vi "Test Open Close.vi"(8 "error in (no error)":errorcluster, 11 "Instrument.Oxford1820 in":refnum<class "Instrument.OxfordVRM.lvclass">) -> (0 "error out":errorcluster, 3 "Instrument.Oxford1820 out":refnum<class "Instrument.OxfordVRM.lvclass">)   [LabVIEW 2019, in "Instrument.OxfordVRM.lvclass"]
uses:
  Instrument.OxfordVRM.lvclass
  <instrlib>/Mercury iXX/Public/Libraries/Magnet/Controls/Device (Read).ctl
  <instrlib>/Mercury iXX/Public/Controls/Manufacturing Data.ctl
  <instrlib>/Mercury iXX/Public/Libraries/Magnet/Controls/Signals (Read).ctl
  Instrument.OxfordVRM.lvclass/Instrument.OxfordVRM.ctl
  <instrlib>/Mercury iXX/Public/Libraries/Magnet/Open/Open Magnet Device.vi
  <instrlib>/Mercury iXX/Public/Libraries/Magnet/Configuration/Read/Magnet Device (Read).vi
  <instrlib>/Mercury iXX/Mercury iXX.lvlib
  <instrlib>/Mercury iXX/Public/Libraries/Magnet.lvlib
panel:
  out "Magnet Device Details":T1={"Manufacturing"={"Hardware Version"="", "Firmware Version"="", "Serial Number"=""}, "Nickname"="", "Bipolar Output"="", "String"="SERS", "Current Limit"=0.0, "AtoB"=0.0, "Inductance"=0.0, "Switch Present"="", "Swh Htr Current"=0.0, "SW VLIM"=0.0, "V Trans Time"=0.0, "Magnet PSU Signals"={"Voltage"=0.0, "Current"=0.0, "Current Rate"=0.0, "Field"=0.0, "Field Rate"=0.0, "Persistant Current"=0.0, "Persistant Field"=0.0, "Target Current"=0.0, "Target Field"=0.0, "Target Current Rate"=0.0, "Target Field Rate"=0.0, "Switch Heater Status (SWHT)"="", "Switch Heater Status (SWHN)"=""}, "PSU Action"="SERS", "Status"="", "Level Limit"=0.0, "Temperature Limit"=0.0} {"Temperature Limit" format="%#.1f"; "Level Limit" format="%#.1f"; "V Trans Time" format="%#.1f"; "SW VLIM" format="%#.1f"; "Swh Htr Current" format="%#.1f"; "Inductance" format="%#.1f"; "AtoB" format="%#.1f"; "Current Limit" format="%#.1f"}
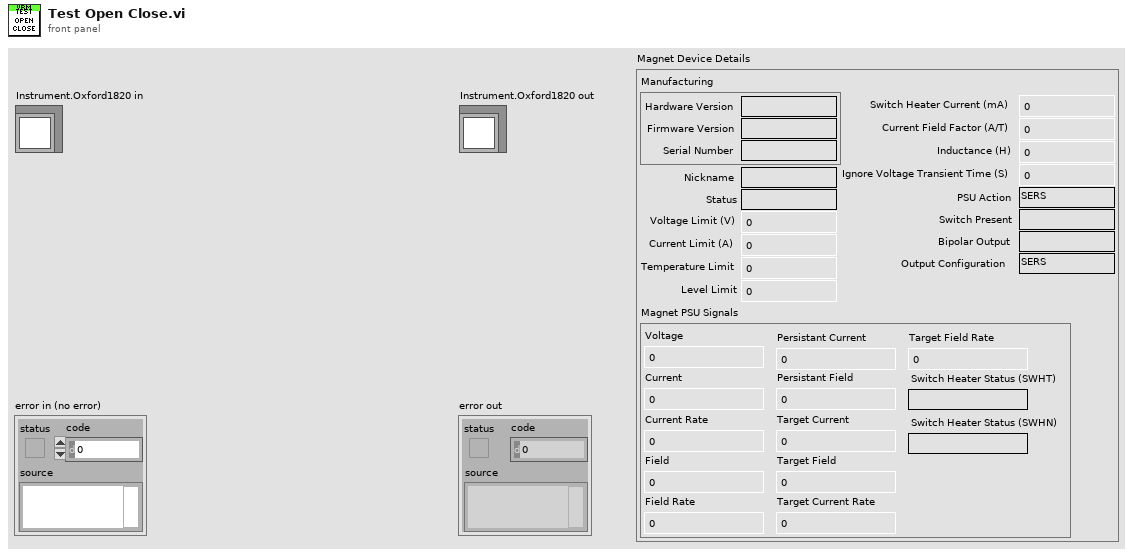
[diagram p1: front panel]
types:
  T1 = typedef "Mercury iXX.lvlib/Magnet.lvlib/Device (Read).ctl" = cluster{"Manufacturing":T2, "Nickname":string, "Bipolar Output":string, "String":string, "Current Limit":dbl, "AtoB":dbl, "Inductance":dbl, "Switch Present":string, "Swh Htr Current":dbl, "SW VLIM":dbl, "V Trans Time":dbl, "Magnet PSU Signals":T3, "PSU Action":string, "Status":string, "Level Limit":dbl, "Temperature Limit":dbl}
  T2 = typedef "Mercury iXX.lvlib/Manufacturing Data.ctl" = cluster{"Hardware Version":string, "Firmware Version":string, "Serial Number":string}
  T3 = typedef "Mercury iXX.lvlib/Magnet.lvlib/Signals (Read).ctl" = cluster{"Voltage":dbl, "Current":dbl, "Current Rate":dbl, "Field":dbl, "Field Rate":dbl, "Persistant Current":dbl, "Persistant Field":dbl, "Target Current":dbl, "Target Field":dbl, "Target Current Rate":dbl, "Target Field Rate":dbl, "Switch Heater Status (SWHT)":string, "Switch Heater Status (SWHN)":string}
  T4 = typedef "Mercury iXX.lvlib/Mercury Reference.ctl" = cluster{"Comms":refnum<visa-resource-name>, "Device ID":string[], "Comms Layer":T5, "Command":string, "Query reference":T6}
  T5 = typedef "Mercury iXX.lvlib/Comms Transport Layer.ctl" = enum16{"Ethernet TCP/IP", "USB", "ISOBus - RS-232", "GPIB"}
  T6 = typedef "Mercury iXX.lvlib/Query Dynamic Reference.ctl" = refnum<vi>
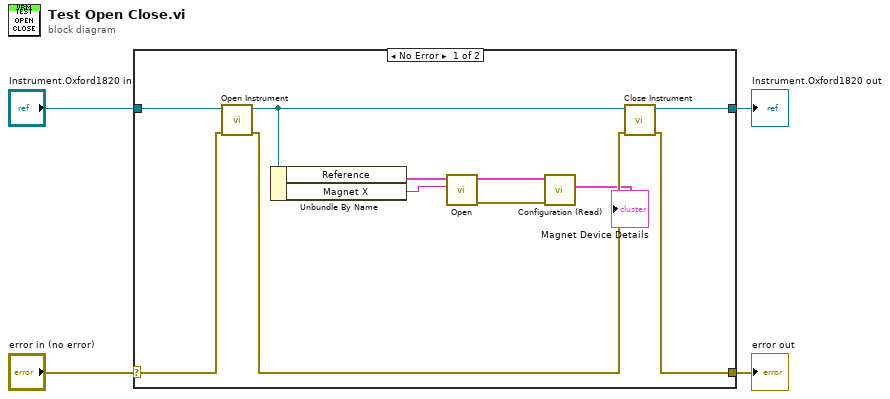
[diagram p0: block diagram]
diagram:
  n1 = case shown="No Error" "error in (no error)" {
    selector: "error in (no error)" -> [w13 w17]
    tunnel: [w11 w17] -> w3
    tunnel: [w14 w16] -> w1
    tunnel: "Instrument.Oxford1820 in" -> [w15 w16]
    frame No Error {
      n2 = call-dynamic "Open Instrument.vi"("error in (no error)"=w13, "Instrument in"=w15) -> ("error out"=w12:errorcluster, "Instrument out"=w10:refnum<class "Instrument.OxfordVRM.lvclass">)  [unwired: 8 in]
      n3 = Unbundle By Name(w10) -> ("Reference"=w9:T4, "Magnet X"=w5:string)
      n4 = call-poly <instrlib>:"Open.vi"("Device Identifier"=w5, "Mercury Reference In"=w9) -> ("error out"=w7:errorcluster, "Mercury Reference Out"=w8:T4)  [unwired: 8 in]
      n5 = call-poly <instrlib>:"Configuration (Read).vi"("error in"=w7, "Mercury Reference In"=w8) -> ("Magnet Device Details"=→"Magnet Device Details":T1)  [unwired: 6 in, 3 out]
      n6 = call-dynamic "Close Instrument.vi"("error in (no error)"=w12, "Instrument in"=w10) -> ("error out"=w11:errorcluster, "Instrument out"=w14:refnum<class "Instrument.OxfordVRM.lvclass">)  [unwired: 8 in]
    }
    frame Error {
    }
  }
  "error out" <- w3
  "Instrument.Oxford1820 out" <- w1
